vi "Update.vi"(8 "error in (no error)":errorcluster, 11 "Main Controller Actor in":refnum<class "Main Controller Actor.lvclass">) -> (0 "error out":errorcluster, 3 "Main Controller Actor out":refnum<class "Main Controller Actor.lvclass">)   [LabVIEW 2021, in "Main Controller Actor.lvclass"]
uses:
  Main Controller Actor.lvclass
  Re-use Libraries/Minimal Actor Framework/Actors/Base Actor/Actor/Actor.lvclass
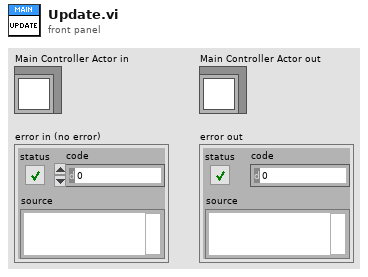
[diagram p1: front panel]
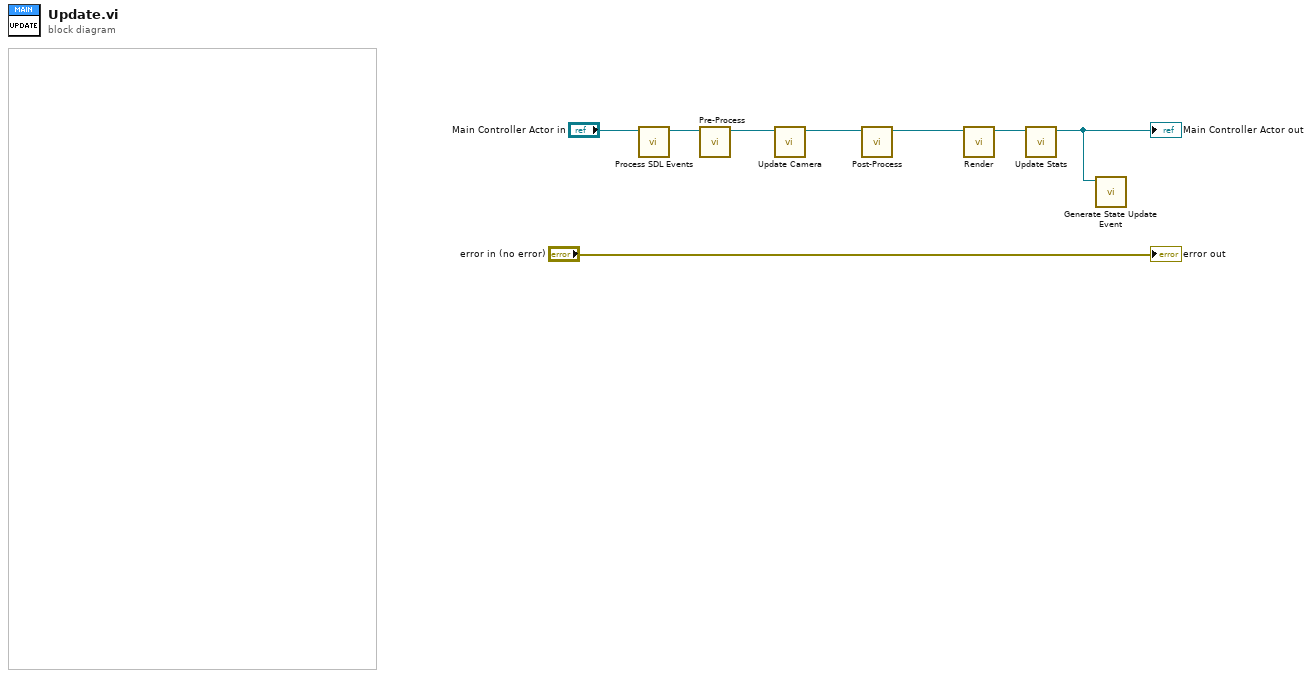
[diagram p0: block diagram]
diagram:
  n1 = call "Process SDL Events.vi"("Main Controller Actor in"="Main Controller Actor in") -> ("Main Controller Actor out"=w5:refnum<class "Main Controller Actor.lvclass">)  [unwired: 10 in]
  n2 = call "Pre-Process.vi"("Main Controller Actor in"=w5) -> ("Main Controller Actor out"=w3:refnum<class "Main Controller Actor.lvclass">)  [unwired: 10 in]
  n3 = call "Update Camera.vi"("Main Controller Actor in"=w3) -> ("Main Controller Actor out"=w2:refnum<class "Main Controller Actor.lvclass">)  [unwired: 10 in]
  n4 = call "Post-Process.vi"("Main Controller Actor in"=w2) -> ("Main Controller Actor out"=w4:refnum<class "Main Controller Actor.lvclass">)  [unwired: 10 in]
  n5 = call "Render.vi"("Main Controller Actor in"=w4) -> ("Main Controller Actor out"=w6:refnum<class "Main Controller Actor.lvclass">)  [unwired: 10 in]
  n6 = call "Update Stats.vi"("Main Controller Actor in"=w6) -> ("Main Controller Actor out"=w1:refnum<class "Main Controller Actor.lvclass">)  [unwired: 10 in]
  "Main Controller Actor out" <- w1
  n7 = call "Generate State Update Event.vi"("Actor in"=w1) -> ()  [unwired: 10 in, 1 out]
  "error out" <- "error in (no error)"
